vi "OnLoad.LegacyLogic.vi"(8 "error in (no error)":errorcluster, 9 "Version Iteration":i32, 10 "Execute?":bool, 11 "Device Ref in":T1 format="%.0x") -> (0 "error out":errorcluster, 3 "Device Ref out":T1 format="%.0x")   [LabVIEW 2023, in "J1939 Addon System Explorer.lvlib"]
uses:
  J1939 Addon System Explorer.lvlib
  <vilib>/NI VeriStand/Custom Device API/Custom Device Item Ref.ctl
  Addon Shared/Types/XNET Settings.ctl
  Addon Shared/Types/Monitor Settings.ctl
  Addon Shared/Types/SPN Properties.ctl
  Addon Shared/SubVIs/Constants.vi
  <vilib>/NI VeriStand/Custom Device API/Get Item Property (Variant).vi
  <vilib>/NI VeriStand/Custom Device Tools/Custom Device Utility Library/NI VeriStand - Search for Item by GUID.vi
  <vilib>/NI VeriStand/Custom Device API/Get Item Property (U16).vi
  <vilib>/NI VeriStand/Custom Device API/Set Item Property (String).vi
  <vilib>/NI VeriStand/Custom Device Tools/Custom Device Utility Library/NI VeriStand - Search for All Items by GUID.vi
  <vilib>/NI VeriStand/Custom Device API/Custom Device API.lvlib
  Addon Shared/J1939 Addon Shared.lvlib
  <vilib>/NI VeriStand/Custom Device Tools/Custom Device Utility Library/Custom Device Utility Library.lvlib
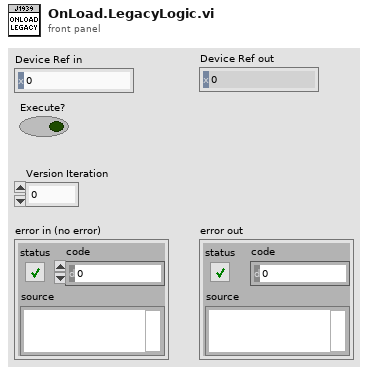
[diagram p1: front panel]
types:
  T1 = typedef "Custom Device API.lvlib/Custom Device Item Ref.ctl" = u64
  T2 = typedef "J1939 Addon Shared.lvlib/Monitor Settings.ctl" = cluster{"Address":u8, "Name":u64, "Include DA":bool, "Force SA":bool}
  T3 = typedef "J1939 Addon Shared.lvlib/XNET Settings.ctl" = cluster{"Database":refnum<k21>, "Cluster":refnum<k21>, "Port":string, "Baud rate [Bd]":u32, "Termination":u32, "Incoming Decimation":u32, "Outgoing Decimation":u32}
  T4 = cluster{"XNET Database":refnum<k21>, "XNET Cluster":refnum<k21>, "CAN Port":string, "Baud rate [Bd]":u32, "J1939 Network Address":u8, "Name":u64, "Termination":u32}
  T5 = cluster{"XNET Database":refnum<k21>, "XNET Cluster":refnum<k21>, "CAN Port":string, "Baud rate [Bd]":u32, "J1939 Network Address":u8, "Name":u64, "Termination":u32, "Incoming Rate":u32, "Outcoming Rate":u32}
  T6 = cluster{"Database":refnum<k21>, "Cluster":refnum<k21>, "Port":string, "Baud rate [Bd]":u32, "Termination":u32, "Incoming Rate":u32, "Outcoming Rate":u32, "Write Decimation":u32}
  T7 = typedef "J1939 Addon Shared.lvlib/SPN Properties.ctl" = cluster{"Bytes":u32, "ScaleFac":dbl, "ScaleOff":dbl}
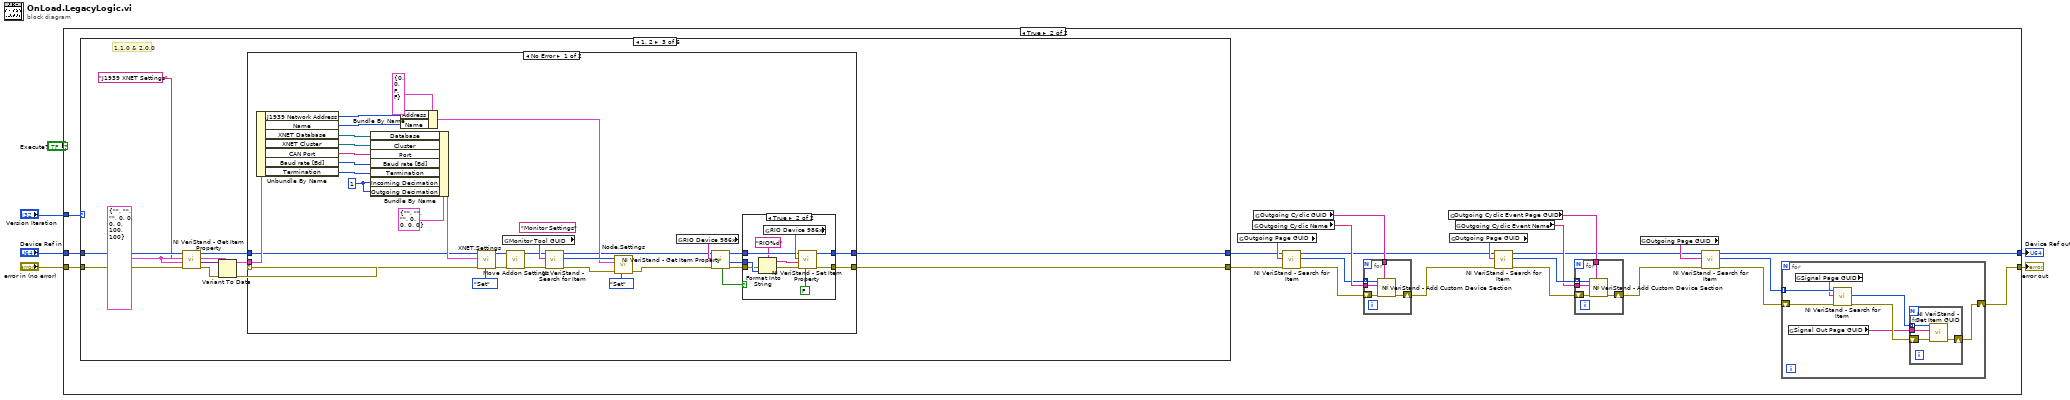
[diagram p0: block diagram]
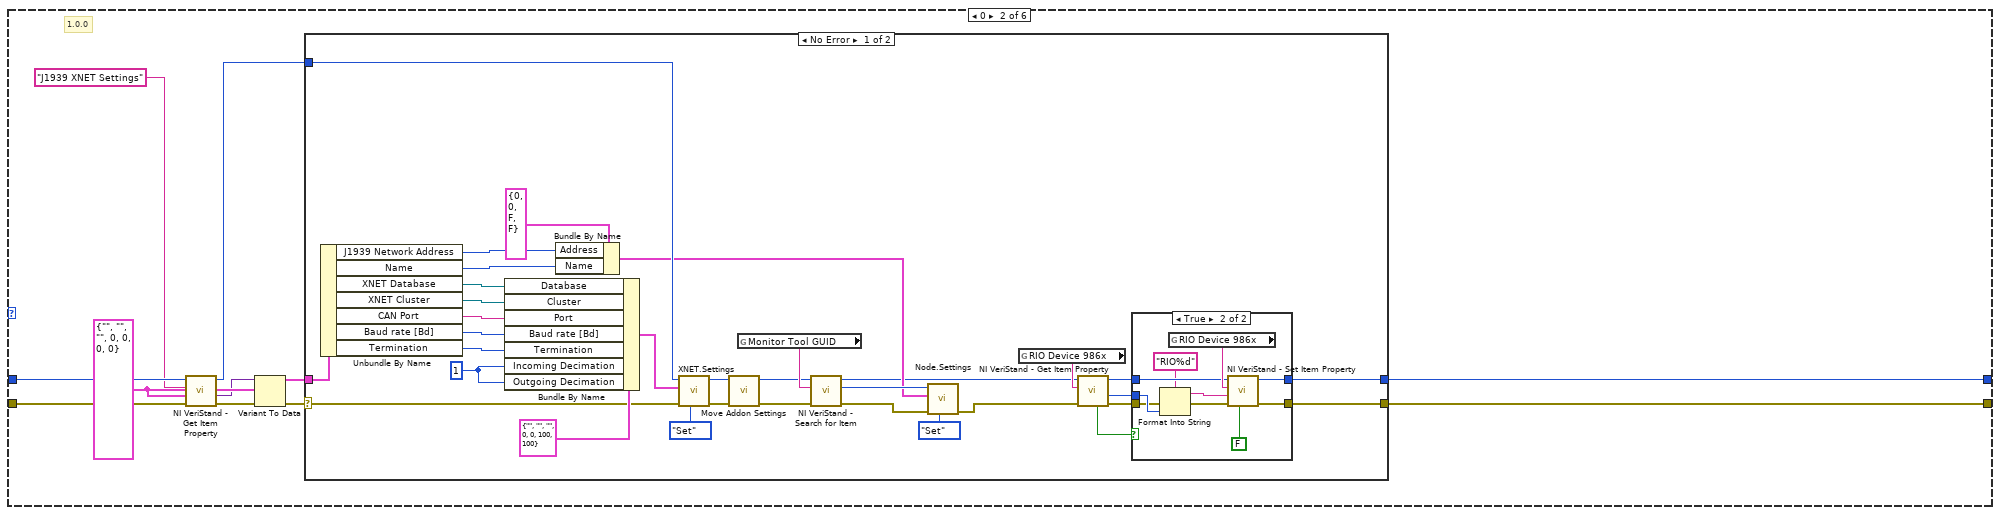
[diagram p4: hidden frame]
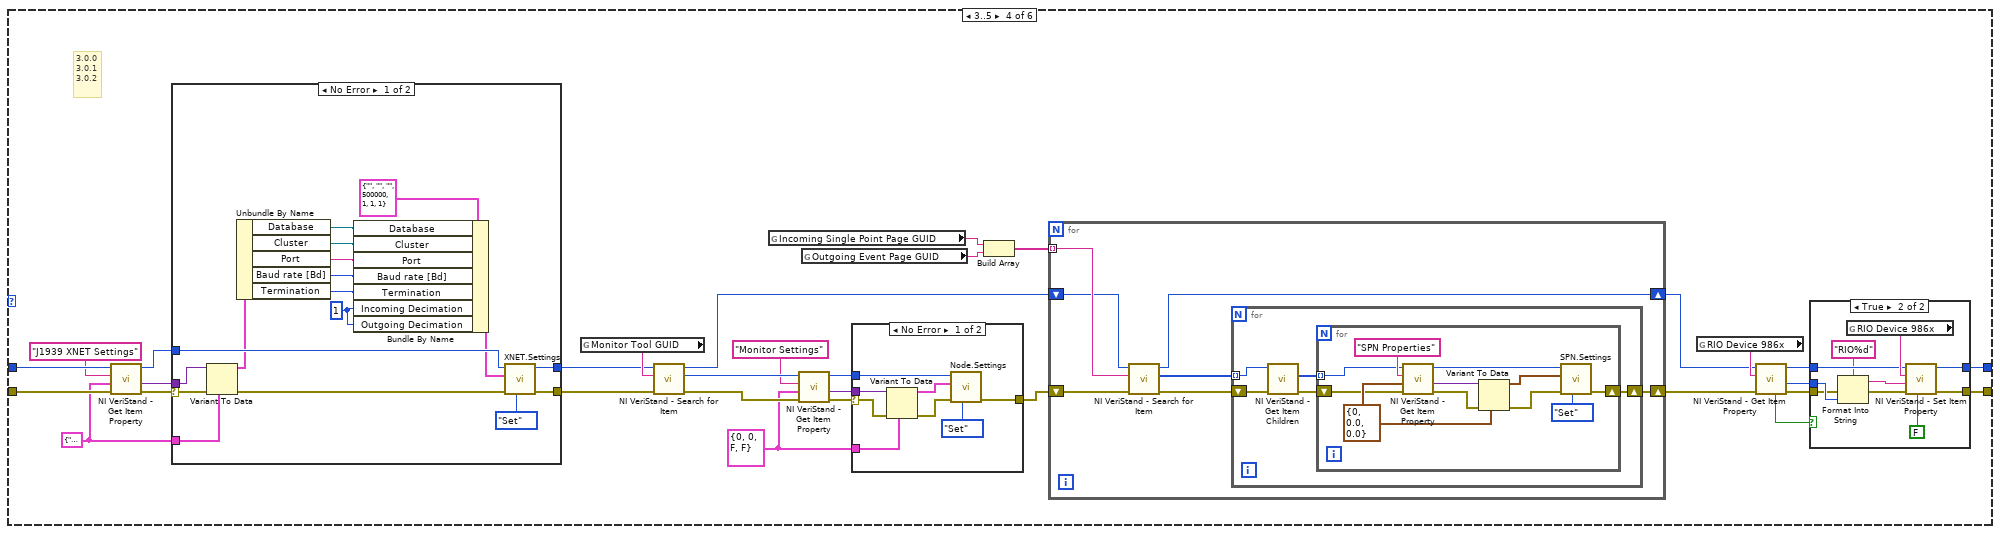
[diagram p9: hidden frame]
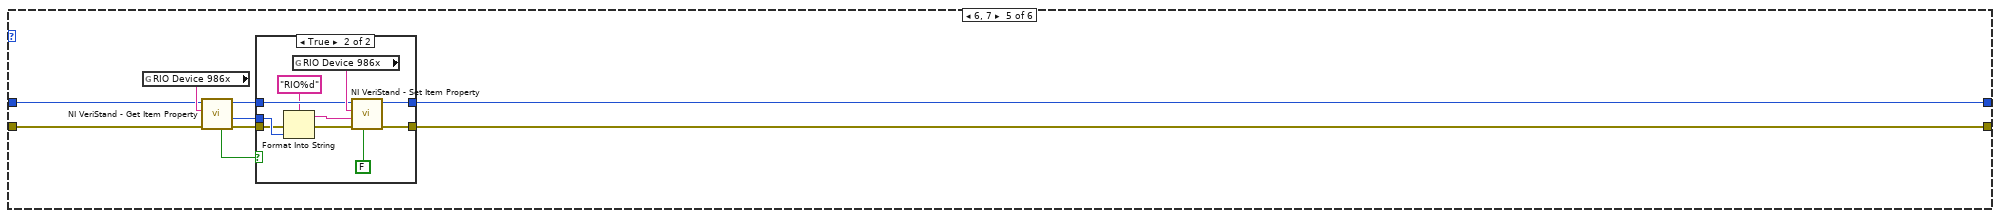
[diagram p13: hidden frame]
diagram:
  n1 = case shown="True" "Execute?" {
    tunnel: "error in (no error)" -> [w8 w32]
    tunnel: [w8 w9] -> w3
    tunnel: "Device Ref in" -> [w7 w30]
    tunnel: [w7 w12] -> w5
    tunnel: "Version Iteration" -> [_ w31]
    frame False {
    }
    frame True {
      n2 = case shown="1, 2" w31 {
        tunnel: w32 -> [w50 w58 w117 w196 w264 w283]
        tunnel: [w50 w54 w113 w168 w262 w283] -> w24
        tunnel: [w49 w53 w112 w167 w261 w282] -> w23
        tunnel: w30 -> [w49 w57 w116 w197 w263 w282]
        frame Default {
        }
        frame 0 {
          w61 = T4 {"XNET Database"="", "XNET Cluster"="", "CAN Port"="", "Baud rate [Bd]"=0, "J1939 Network Address"=0, "Name"=0, "Termination"=0} ("J1939 XNET Settings")
          # "1.0.0"
          n3 = call-poly <vilib>:"NI VeriStand - Get Item Property.vi"("error in (no error)"=w58, "Default Value"=w61, "Property Name"="J1939 XNET Settings" ("J1939 XNET Settings"), "Item Ref in"=w57) -> ("error out"=w59:errorcluster, "Value"=w60:variant, "Item Ref out"=w55:T1)  [unwired: 4 in, 1 out]
          n4 = Variant To Data(error in=w59, type=w61, Variant=w60) -> (data=w56:T4, error out=w52:errorcluster)
          n5 = case shown="No Error" w52 {
            selector: w52 -> [w87 w107]
            tunnel: w56 -> [w94 _]
            tunnel: w55 -> [w88 w108]
            tunnel: [w66 w107] -> w54
            tunnel: [w62 w108] -> w53
            frame No Error {
              w80 = u32 1 ("Incoming Rate")
              n6 = Unbundle By Name(w94) -> ("J1939 Network Address"=w82:u8, "Name"=w83:u64, "XNET Database"=w92:refnum<k21>, "XNET Cluster"=w91:refnum<k21>, "CAN Port"=w90:string, "Baud rate [Bd]"=w89:u32, "Termination"=w85:u32)
              n7 = Bundle By Name(cluster=T3 {"Database"="", "Cluster"="", "Port"="", "Baud rate [Bd]"=0, "Termination"=0, "Incoming Decimation"=100, "Outgoing Decimation"=100} ("J1939 XNET Settings"), "Database"=w92, "Cluster"=w91, "Port"=w90, "Baud rate [Bd]"=w89, "Termination"=w85, "Incoming Decimation"=w80, "Outgoing Decimation"=w80) -> (w74:T3)
              n8 = Bundle By Name(cluster=T2 {"Address"=0, "Name"=0, "Include DA"=FALSE, "Force SA"=FALSE} ("J1939 Monitor Settings"), "Address"=w82, "Name"=w83) -> (w72:T2)
              n9 = call "XNET.Settings.vi"("Action"=enum8{"Get", "Set"}."Set", "error in (no error)"=w87, "J1939 XNET Settings"=w74, "Parent Ref in"=w88) -> ("error out"=w76:errorcluster, "Item Ref out"=w78:T1)  [unwired: 5 in, 1 out]
              n10 = call "Move Addon Settings.vi"("error in (no error)"=w76, "Section Ref in"=w78) -> ("error out"=w75:errorcluster, "Parent Ref out"=w77:T1)  [unwired: 8 in]
              n11 = global read "Constants.vi" "Monitor Tool GUID"() -> (w86:string)
              n12 = call-poly <vilib>:"NI VeriStand - Search for Item.vi"("error in"=w75, "Item GUID"=w86, "Section Ref in"=w77) -> ("error out"=w81:errorcluster, "Item Ref"=w79:T1, "Section Ref out"=w63:T1)  [unwired: 5 in, 1 out]
              n13 = call "Node.Settings.vi"("Action"=enum8{"Get", "Set"}."Set", "error in (no error)"=w81, "Node.Settings"=w72, "Item Ref in"=w79) -> ("error out"=w69:errorcluster)  [unwired: 5 in, 2 out]
              n14 = global read "Constants.vi" "RIO Device 986x"() -> (w70:string)
              n15 = call-poly <vilib>:"NI VeriStand - Get Item Property.vi"("error in (no error)"=w69, "Property Name"=w70, "Item Ref in"=w63) -> ("error out"=w67:errorcluster, "Value"=w64:u16, "Item Ref out"=w68:T1, "Found?"=w65:bool)  [unwired: 5 in]
              n16 = case shown="True" w65 {
                tunnel: w68 -> [w95 w105]
                tunnel: w67 -> [w96 w101]
                tunnel: [w96 w104] -> w66
                tunnel: w64 -> [_ w102]
                tunnel: [w95 w98] -> w62
                frame False {
                }
                frame True {
                  n17 = Format Into String(format string="RIO%d", error in=w101, w102) -> (resulting string=w97:string, error out=w100:errorcluster)  [unwired: 1 in]
                  n18 = global read "Constants.vi" "RIO Device 986x"() -> (w106:string)
                  n19 = call-poly <vilib>:"NI VeriStand - Set Item Property.vi"("Binary String (T)"=FALSE ("Replaced"), "error in (no error)"=w100, "Value"=w97, "Property Name"=w106, "Item Ref in"=w105) -> ("error out"=w104:errorcluster, "Item Ref out"=w98:T1)  [unwired: 4 in, 1 out]
                }
              }
            }
            frame Error {
            }
          }
        }
        frame 1, 2 {
          w110 = T5 {"XNET Database"="", "XNET Cluster"="", "CAN Port"="", "Baud rate [Bd]"=0, "J1939 Network Address"=0, "Name"=0, "Termination"=0, "Incoming Rate"=100, "Outcoming Rate"=100} ("J1939 XNET Settings")
          # "1.1.0 & 2.0.0"
          n20 = call-poly <vilib>:"NI VeriStand - Get Item Property.vi"("error in (no error)"=w117, "Default Value"=w110, "Property Name"="J1939 XNET Settings" ("J1939 XNET Settings"), "Item Ref in"=w116) -> ("error out"=w118:errorcluster, "Value"=w119:variant, "Item Ref out"=w114:T1)  [unwired: 4 in, 1 out]
          n21 = Variant To Data(error in=w118, type=w110, Variant=w119) -> (data=w115:T5, error out=w111:errorcluster)
          n22 = case shown="No Error" w111 {
            selector: w111 -> [w131 w165]
            tunnel: w115 -> [w152 _]
            tunnel: w114 -> [w130 w166]
            tunnel: [w122 w165] -> w113
            tunnel: [w120 w166] -> w112
            frame No Error {
              w129 = u32 1 ("Incoming Decimation")
              (unwired) "Monitor Settings" ("J1939 Monitor Settings")
              n23 = Unbundle By Name(w152) -> ("J1939 Network Address"=w142:u8, "Name"=w143:u64, "XNET Database"=w150:refnum<k21>, "XNET Cluster"=w149:refnum<k21>, "CAN Port"=w148:string, "Baud rate [Bd]"=w147:u32, "Termination"=w145:u32)
              n24 = Bundle By Name(cluster=T3 {"Database"="", "Cluster"="", "Port"="", "Baud rate [Bd]"=0, "Termination"=0, "Incoming Decimation"=0, "Outgoing Decimation"=0} ("J1939 XNET Settings"), "Database"=w150, "Cluster"=w149, "Port"=w148, "Baud rate [Bd]"=w147, "Termination"=w145, "Incoming Decimation"=w129, "Outgoing Decimation"=w129) -> (w135:T3)
              n25 = Bundle By Name(cluster=T2 {"Address"=0, "Name"=0, "Include DA"=FALSE, "Force SA"=FALSE} ("J1939 Monitor Settings"), "Address"=w142, "Name"=w143) -> (w134:T2)
              n26 = call "XNET.Settings.vi"("Action"=enum8{"Get", "Set"}."Set", "error in (no error)"=w131, "J1939 XNET Settings"=w135, "Parent Ref in"=w130) -> ("error out"=w137:errorcluster, "Item Ref out"=w139:T1)  [unwired: 5 in, 1 out]
              n27 = global read "Constants.vi" "Monitor Tool GUID"() -> (w146:string)
              n28 = call "Move Addon Settings.vi"("error in (no error)"=w137, "Section Ref in"=w139) -> ("error out"=w136:errorcluster, "Parent Ref out"=w138:T1)  [unwired: 8 in]
              n29 = call-poly <vilib>:"NI VeriStand - Search for Item.vi"("error in"=w136, "Item GUID"=w146, "Section Ref in"=w138) -> ("error out"=w141:errorcluster, "Item Ref"=w140:T1, "Section Ref out"=w121:T1)  [unwired: 5 in, 1 out]
              n30 = call "Node.Settings.vi"("Action"=enum8{"Get", "Set"}."Set", "error in (no error)"=w141, "Node.Settings"=w134, "Item Ref in"=w140) -> ("error out"=w123:errorcluster)  [unwired: 5 in, 2 out]
              n31 = global read "Constants.vi" "RIO Device 986x"() -> (w128:string)
              n32 = call-poly <vilib>:"NI VeriStand - Get Item Property.vi"("error in (no error)"=w123, "Property Name"=w128, "Item Ref in"=w121) -> ("error out"=w126:errorcluster, "Value"=w124:u16, "Item Ref out"=w127:T1, "Found?"=w125:bool)  [unwired: 5 in]
              n33 = case shown="True" w125 {
                tunnel: w127 -> [w153 w163]
                tunnel: w126 -> [w154 w159]
                tunnel: [w154 w162] -> w122
                tunnel: w124 -> [_ w160]
                tunnel: [w153 w156] -> w120
                frame False {
                }
                frame True {
                  n34 = Format Into String(format string="RIO%d", error in=w159, w160) -> (resulting string=w155:string, error out=w158:errorcluster)  [unwired: 1 in]
                  n35 = global read "Constants.vi" "RIO Device 986x"() -> (w164:string)
                  n36 = call-poly <vilib>:"NI VeriStand - Set Item Property.vi"("Binary String (T)"=FALSE ("Replaced"), "error in (no error)"=w158, "Value"=w155, "Property Name"=w164, "Item Ref in"=w163) -> ("error out"=w162:errorcluster, "Item Ref out"=w156:T1)  [unwired: 4 in, 1 out]
                }
              }
            }
            frame Error {
            }
          }
        }
        frame 3..5 {
          w181 = T2 {"Address"=0, "Name"=0, "Include DA"=FALSE, "Force SA"=FALSE} ("J1939 Monitor Settings")
          w192 = T6 {"Database"="", "Cluster"="", "Port"="", "Baud rate [Bd]"=0, "Termination"=0, "Incoming Rate"=0, "Outcoming Rate"=0, "Write Decimation"=0} ("J1939 XNET Settings")
          # "3.0.0\n3.0.1\n3.0.2"
          n37 = call-poly <vilib>:"NI VeriStand - Get Item Property.vi"("error in (no error)"=w196, "Default Value"=w192, "Property Name"="J1939 XNET Settings" ("J1939 XNET Settings"), "Item Ref in"=w197) -> ("error out"=w194:errorcluster, "Value"=w193:variant, "Item Ref out"=w191:T1)  [unwired: 4 in, 1 out]
          n38 = case shown="No Error" w194 {
            selector: w194 -> [w226 w228]
            tunnel: w193 -> [w225 _]
            tunnel: w192 -> [w224 _]
            tunnel: w191 -> [w221 w227]
            tunnel: [w220 w227] -> w188
            tunnel: [w219 w228] -> w189
            frame No Error {
              w210 = u32 1 ("Incoming Decimation")
              n39 = Variant To Data(error in=w226, type=w224, Variant=w225) -> (data=w216:T6, error out=w222:errorcluster)
              n40 = Unbundle By Name(w216) -> ("Database"=w215:refnum<k21>, "Cluster"=w211:refnum<k21>, "Port"=w212:string, "Baud rate [Bd]"=w213:u32, "Termination"=w214:u32)
              n41 = Bundle By Name(cluster=T3 {"Database"="", "Cluster"="", "Port"="", "Baud rate [Bd]"=500000, "Termination"=1, "Incoming Decimation"=1, "Outgoing Decimation"=1} ("J1939 XNET Settings"), "Database"=w215, "Cluster"=w211, "Port"=w212, "Baud rate [Bd]"=w213, "Termination"=w214, "Incoming Decimation"=w210, "Outgoing Decimation"=w210) -> (w217:T3)
              n42 = call "XNET.Settings.vi"("Action"=enum8{"Get", "Set"}."Set", "error in (no error)"=w222, "J1939 XNET Settings"=w217, "Parent Ref in"=w221) -> ("error out"=w219:errorcluster, "Item Ref out"=w220:T1)  [unwired: 5 in, 1 out]
            }
            frame Error {
            }
          }
          n43 = global read "Constants.vi" "Monitor Tool GUID"() -> (w190:string)
          n44 = call-poly <vilib>:"NI VeriStand - Search for Item.vi"("error in"=w189, "Item GUID"=w190, "Section Ref in"=w188) -> ("error out"=w187:errorcluster, "Item Ref"=w186:T1, "Section Ref out"=w176:T1)  [unwired: 5 in, 1 out]
          n45 = global read "Constants.vi" "Incoming Single Point Page GUID"() -> (w179:string)
          n46 = call-poly <vilib>:"NI VeriStand - Get Item Property.vi"("error in (no error)"=w187, "Default Value"=w181, "Property Name"="Monitor Settings" ("J1939 Monitor Settings"), "Item Ref in"=w186) -> ("error out"=w182:errorcluster, "Value"=w183:variant, "Item Ref out"=w184:T1)  [unwired: 4 in, 1 out]
          n47 = global read "Constants.vi" "Outgoing Event Page GUID"() -> (w178:string)
          n48 = case shown="No Error" w182 {
            selector: w182 -> [w259 w260]
            tunnel: w183 -> [w258 _]
            tunnel: w181 -> [w257 _]
            tunnel: w184 -> [w254 _]
            tunnel: [w253 w260] -> w177
            frame No Error {
              n49 = Variant To Data(error in=w259, type=w257, Variant=w258) -> (data=w252:T2, error out=w255:errorcluster)
              n50 = call "Node.Settings.vi"("Action"=enum8{"Get", "Set"}."Set", "error in (no error)"=w255, "Node.Settings"=w252, "Item Ref in"=w254) -> ("error out"=w253:errorcluster)  [unwired: 5 in, 2 out]
            }
            frame Error {
            }
          }
          n51 = Build Array(w179, w178) -> (w180:string[])
          n52 = for {
            tunnel: w180 -> [w235] mode=indexing
            shift-right: [w232] -> w170
            shift-left: w177 -> [w231]
            shift-right: [w230] -> w169
            shift-left: w176 -> [w229]
            n53 = call-poly <vilib>:"NI VeriStand - Search for Item.vi"("error in"=w231, "Item GUID"=w235, "Section Ref in"=w229) -> ("error out"=w233:errorcluster, "Item Refs"=w234:T1[], "Section Ref out"=w230:T1)  [unwired: 5 in, 1 out]
            n54 = for {
              tunnel: w234 -> [w239] mode=indexing
              shift-right: [w236] -> w232
              shift-left: w233 -> [w240]
              n55 = call <vilib>:"NI VeriStand - Get Item Children.vi"("error in (no error)"=w240, "Item Ref in"=w239) -> ("error out"=w237:errorcluster, "Child Refs"=w238:T1[])  [unwired: 6 in, 2 out]
              n56 = for {
                tunnel: w238 -> [w246] mode=indexing
                shift-right: [w242] -> w236
                shift-left: w237 -> [w247]
                w250 = T7 {"Bytes"=0, "ScaleFac"=0.0, "ScaleOff"=0.0} ("cluster")
                n57 = call-poly <vilib>:"NI VeriStand - Get Item Property.vi"("error in (no error)"=w247, "Default Value"=w250, "Property Name"="SPN Properties" ("SPN Properties"), "Item Ref in"=w246) -> ("error out"=w249:errorcluster, "Value"=w248:variant, "Item Ref out"=w245:T1)  [unwired: 4 in, 1 out]
                n58 = Variant To Data(error in=w249, type=w250, Variant=w248) -> (data=w244:T7, error out=w243:errorcluster)
                n59 = call "SPN.Settings.vi"("Action"=enum8{"Get", "Set"}."Set", "error in (no error)"=w243, "SPN.Settings"=w244, "Item Ref in"=w245) -> ("error out"=w242:errorcluster)  [unwired: 5 in, 2 out]
              }
            }
          }
          n60 = global read "Constants.vi" "RIO Device 986x"() -> (w175:string)
          n61 = call-poly <vilib>:"NI VeriStand - Get Item Property.vi"("error in (no error)"=w170, "Property Name"=w175, "Item Ref in"=w169) -> ("error out"=w173:errorcluster, "Value"=w171:u16, "Item Ref out"=w174:T1, "Found?"=w172:bool)  [unwired: 5 in]
          n62 = case shown="True" w172 {
            tunnel: w174 -> [w198 w208]
            tunnel: w173 -> [w199 w204]
            tunnel: [w199 w207] -> w168
            tunnel: w171 -> [_ w205]
            tunnel: [w198 w201] -> w167
            frame False {
            }
            frame True {
              n63 = Format Into String(format string="RIO%d", error in=w204, w205) -> (resulting string=w200:string, error out=w203:errorcluster)  [unwired: 1 in]
              n64 = global read "Constants.vi" "RIO Device 986x"() -> (w209:string)
              n65 = call-poly <vilib>:"NI VeriStand - Set Item Property.vi"("Binary String (T)"=FALSE ("Replaced"), "error in (no error)"=w203, "Value"=w200, "Property Name"=w209, "Item Ref in"=w208) -> ("error out"=w207:errorcluster, "Item Ref out"=w201:T1)  [unwired: 4 in, 1 out]
            }
          }
        }
        frame 6, 7 {
          n66 = global read "Constants.vi" "RIO Device 986x"() -> (w269:string)
          n67 = call-poly <vilib>:"NI VeriStand - Get Item Property.vi"("error in (no error)"=w264, "Property Name"=w269, "Item Ref in"=w263) -> ("error out"=w267:errorcluster, "Value"=w265:u16, "Item Ref out"=w268:T1, "Found?"=w266:bool)  [unwired: 5 in]
          n68 = case shown="True" w266 {
            tunnel: w268 -> [w270 w280]
            tunnel: w267 -> [w271 w276]
            tunnel: [w271 w279] -> w262
            tunnel: w265 -> [_ w277]
            tunnel: [w270 w273] -> w261
            frame False {
            }
            frame True {
              n69 = Format Into String(format string="RIO%d", error in=w276, w277) -> (resulting string=w272:string, error out=w275:errorcluster)  [unwired: 1 in]
              n70 = global read "Constants.vi" "RIO Device 986x"() -> (w281:string)
              n71 = call-poly <vilib>:"NI VeriStand - Set Item Property.vi"("Binary String (T)"=FALSE ("Replaced"), "error in (no error)"=w275, "Value"=w272, "Property Name"=w281, "Item Ref in"=w280) -> ("error out"=w279:errorcluster, "Item Ref out"=w273:T1)  [unwired: 4 in, 1 out]
            }
          }
        }
        frame 8..10 {
        }
      }
      n72 = global read "Constants.vi" "Outgoing Page GUID"() -> (w29:string)
      n73 = global read "Constants.vi" "Outgoing Cyclic Name"() -> (w27:string)
      n74 = global read "Constants.vi" "Outgoing Cyclic GUID"() -> (w28:string)
      n75 = call-poly <vilib>:"NI VeriStand - Search for Item.vi"("error in"=w24, "Item GUID"=w29, "Section Ref in"=w23) -> ("error out"=w25:errorcluster, "Item Refs"=w26:T1[], "Section Ref out"=w16:T1)  [unwired: 5 in, 1 out]
      n76 = for {
        tunnel: w28 -> [w288]
        tunnel: w27 -> [w287]
        tunnel: w26 -> [w286] mode=indexing
        shift-right: [w284] -> w17
        shift-left: w25 -> [w285]
        n77 = call <vilib>:"NI VeriStand - Add Custom Device Section.vi"("GUID (Default Section)"=w288, "error in (no error)"=w285, "Section Name"=w287, "Parent Ref in"=w286) -> ("error out"=w284:errorcluster)  [unwired: 4 in, 3 out]
      }
      n78 = global read "Constants.vi" "Outgoing Cyclic Event Page GUID"() -> (w19:string)
      n79 = global read "Constants.vi" "Outgoing Page GUID"() -> (w18:string)
      n80 = global read "Constants.vi" "Outgoing Cyclic Event Name"() -> (w20:string)
      n81 = call-poly <vilib>:"NI VeriStand - Search for Item.vi"("error in"=w17, "Item GUID"=w18, "Section Ref in"=w16) -> ("error out"=w22:errorcluster, "Item Refs"=w21:T1[], "Section Ref out"=w13:T1)  [unwired: 5 in, 1 out]
      n82 = for {
        tunnel: w19 -> [w48]
        tunnel: w20 -> [w47]
        tunnel: w21 -> [w46] mode=indexing
        shift-right: [w44] -> w14
        shift-left: w22 -> [w45]
        n83 = call <vilib>:"NI VeriStand - Add Custom Device Section.vi"("GUID (Default Section)"=w48, "error in (no error)"=w45, "Section Name"=w47, "Parent Ref in"=w46) -> ("error out"=w44:errorcluster)  [unwired: 4 in, 3 out]
      }
      n84 = global read "Constants.vi" "Outgoing Page GUID"() -> (w15:string)
      n85 = call-poly <vilib>:"NI VeriStand - Search for Item.vi"("error in"=w14, "Item GUID"=w15, "Section Ref in"=w13) -> ("error out"=w10:errorcluster, "Item Refs"=w11:T1[], "Section Ref out"=w12:T1)  [unwired: 5 in, 1 out]
      n86 = for {
        tunnel: w11 -> [w39] mode=indexing
        shift-right: [w34] -> w9
        shift-left: w10 -> [w37]
        n87 = global read "Constants.vi" "Signal Out Page GUID"() -> (w33:string)
        n88 = global read "Constants.vi" "Signal Page GUID"() -> (w38:string)
        n89 = call-poly <vilib>:"NI VeriStand - Search for Item.vi"("error in"=w37, "Item GUID"=w38, "Section Ref in"=w39) -> ("error out"=w35:errorcluster, "Item Refs"=w36:T1[])  [unwired: 5 in, 2 out]
        n90 = for {
          tunnel: w36 -> [w43] mode=indexing
          shift-right: [w41] -> w34
          shift-left: w35 -> [w42]
          tunnel: w33 -> [w40]
          n91 = call <vilib>:"NI VeriStand - Set Item GUID.vi"("error in (no error)"=w42, "GUID"=w40, "Item Ref in"=w43) -> ("error out"=w41:errorcluster)  [unwired: 7 in, 1 out]
        }
      }
    }
  }
  "Device Ref out" <- w5
  "error out" <- w3
